vi "5. Write and Read Configuration.vi"() -> ()   [LabVIEW 2017]
uses:
  290c8616-03bb-43f6-9755-f4108a778465.vi
  eb649152-3eda-4c32-aea1-608038e9a66f.vi
  fab2b0d5-8214-42e3-87d5-297c1f02bb71.vi
  13992e20-2d4c-4375-bad9-897eae809fc0.vi
  79b73396-53b7-4374-b6a7-04cba797c1a6.vi
  290c8616-03bb-43f6-9755-f4108a778465.vi/99de0c97-112a-4c86-9094-c187659127e1.vi
  <vilib>/Utility/error.llb/Clear Errors.vi
  eb649152-3eda-4c32-aea1-608038e9a66f.vi/b09b9099-6be0-413b-8afc-4908471460c3.vi
  fab2b0d5-8214-42e3-87d5-297c1f02bb71.vi/b09b9099-6be0-413b-8afc-4908471460c3.vi
  13992e20-2d4c-4375-bad9-897eae809fc0.vi/99de0c97-112a-4c86-9094-c187659127e1.vi
  <userlib>/_NEVSTOP/Communicable State Machine(CSM)/Utility/Build Error Cluster.vi
  79b73396-53b7-4374-b6a7-04cba797c1a6.vi/99de0c97-112a-4c86-9094-c187659127e1.vi
  <vilib>/Utility/Data Type/Get Type Information.vi
  <userlib>/_NEVSTOP/Communicable State Machine(CSM)/addons/API-String-Arugments-Support/_Support/Data To SingleElementsArray_csm.vi
  <userlib>/_NEVSTOP/Communicable State Machine(CSM)/addons/API-String-Arugments-Support/_Support/Data To API String Arguments.vi
  INI-Static-Variable-Support/_Support/Parse Used Session and Name.vi
  INI-Static-Variable-Support/_Support/INI-FGV(lvlibp).vi
  INI-Static-Variable-Support/_Support/Populate String with INI Variable.vi
  <userlib>/_NEVSTOP/Communicable State Machine(CSM)/addons/API-String-Arugments-Support/_Support/Convert API String Arguments to Data(variant).vi
  <userlib>/_NEVSTOP/Communicable State Machine(CSM)/addons/API-String-Arugments-Support/_Support/SingleElementsArray To Data_csm.vi
  INI-Static-Variable-Support/_Support/global-csm-ini-db-change-flag.vi
  INI-Static-Variable-Support/INI-Static-Variable-Support.lvlib
panel:
  out "ip only":cluster{"ip":string}={"ip"="10.144.41.41"}
  out "existing section 2":cluster{"ip":string, "port":i32}={"ip"="10.144.41.41", "port"=8080}
  out "existing section":cluster{"ip":string, "port":i32}={"ip"="10.144.41.41", "port"=8080}
  out "non-existing section":cluster{"ip":string, "port":i32}={"ip"="127.0.0.1", "port"=80}
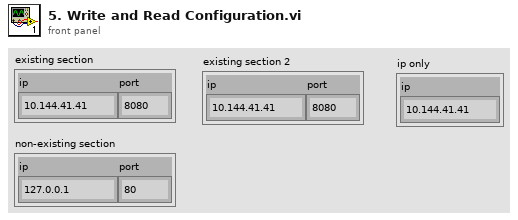
[diagram p1: front panel]
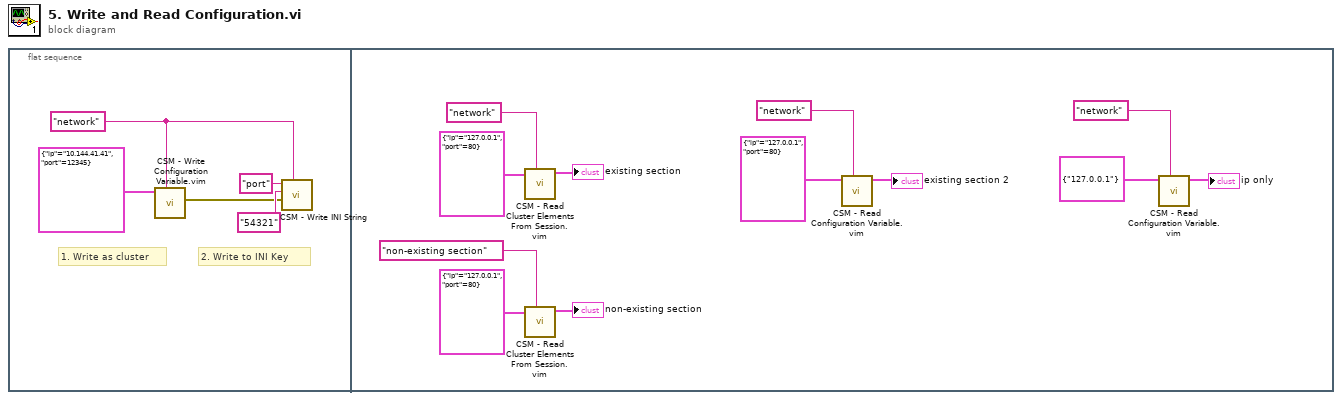
[diagram p0: block diagram]
diagram:
  n1 = flat-sequence {
    frame #0 {
      w4 = "network" ("Section Name(\"\" as Default)")
      # "2. Write to INI Key"
      # "1. Write as cluster"
      n2 = call "CSM - Write Configuration Variable.vim"("Section Name(\"\" as Default)"=w4, "Variant"=cluster{"ip":string, "port":i32} {"ip"="10.144.41.41", "port"=12345}) -> ("error out"=w1:errorcluster)  [unwired: 6 in, 1 out]
      n3 = call "CSM - Write INI String.vi"("Section Name(\"\" as Default)"=w4, "error in (no error)"=w1, "String"="54321", ">> Variable Name >>"="port") -> ()  [unwired: 4 in, 2 out]
    }
    frame #1 {
      n4 = call "CSM - Read Cluster Elements From Session.vim"("Section Name(\"\" as Default)"="network" ("Section Name(\"\" as Default)"), "Cluster"=cluster{"ip":string, "port":i32} {"ip"="127.0.0.1", "port"=80}) -> ("Cluster out"=→"existing section":cluster{"ip":string, "port":i32})  [unwired: 6 in, 1 out]
      n5 = call "CSM - Read Cluster Elements From Session.vim"("Section Name(\"\" as Default)"="non-existing section" ("Section Name(\"\" as Default)"), "Cluster"=cluster{"ip":string, "port":i32} {"ip"="127.0.0.1", "port"=80}) -> ("Cluster out"=→"non-existing section":cluster{"ip":string, "port":i32})  [unwired: 6 in, 1 out]
      n6 = call "CSM - Read Configuration Variable.vim"("Section Name(\"\" as Default)"="network" ("Section Name(\"\" as Default)"), "config prototype(Cluster Prefered)"=cluster{"ip":string, "port":i32} {"ip"="127.0.0.1", "port"=80}) -> ("config out"=→"existing section 2":cluster{"ip":string, "port":i32})  [unwired: 6 in, 1 out]
      n7 = call "CSM - Read Configuration Variable.vim"("Section Name(\"\" as Default)"="network" ("Section Name(\"\" as Default)"), "config prototype(Cluster Prefered)"=cluster{"ip":string} {"ip"="127.0.0.1"}) -> ("config out"=→"ip only":cluster{"ip":string})  [unwired: 6 in, 1 out]
    }
  }
